vi "Replace GUIDs in Constants VI.vi"(8 "error in":errorcluster, 10 "guid map":map{string, string}(c390), 11 "VI in":refnum<vi>) -> (0 "error out":errorcluster, 3 "VI out":refnum<vi>)   [LabVIEW 2020, in "Utility.lvlib"]
uses:
  Utility.lvlib
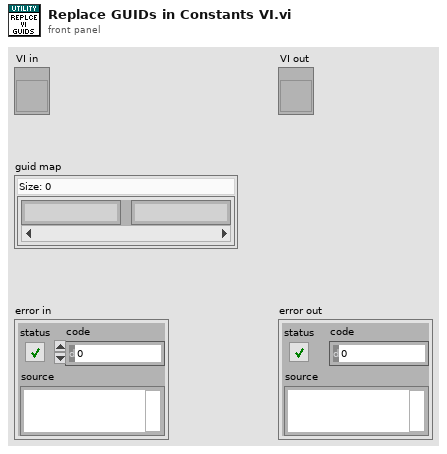
[diagram p1: front panel]
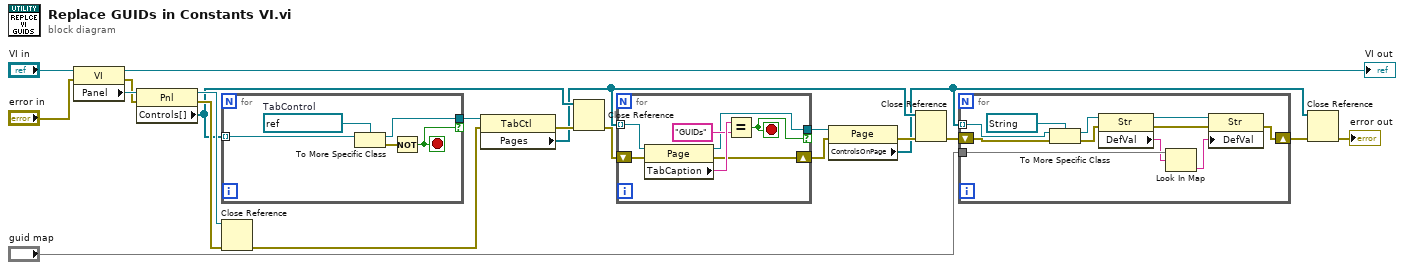
[diagram p0: block diagram]
diagram:
  n1 = property class="VI"(reference="VI in", error in="error in") -> (reference out=→"VI out":refnum<vi>, error out=w15:errorcluster, "Panel"=w19:refnum<vi>)
  n2 = property class="Pnl"(reference=w19, error in=w15) -> (reference out=w13:refnum<vi>, error out=w14:errorcluster, "Controls[]"=w5:refnum<vi>[])
  n3 = for {
    tunnel: w5 -> [w26] mode=indexing
    tunnel: [w24] -> w20 if=w22
    stop <- w22 stop-if-true
    w25 = refnum<vi> refnum  # TabControl
    n4 = To More Specific Class(target class=w25, reference=w26) -> (specific class reference=w24:refnum<vi>, error out=w23:errorcluster)  [unwired: 1 in]
    n5 = Not(x=w23) -> (.not. x?=w22:bool)
  }
  n6 = Close Reference(reference=w13, error in (no error)=w14) -> (error out=w12:errorcluster)
  n7 = property class="TabCtl"(reference=w20, error in=w12) -> (error out=w11:errorcluster, "Pages"=w3:refnum<vi>[])  [unwired: 1 out]
  n8 = Close Reference(reference=w5, error in (no error)=w11) -> (error out=w6:errorcluster)
  n9 = for {
    tunnel: w3 -> [w33] mode=indexing
    tunnel: [w30] -> w21 if=w29
    shift-right: [w27] -> w10
    shift-left: w6 -> [w28]
    stop <- w29 stop-if-true
    n10 = property class="Page"(reference=w33, error in=w28) -> (reference out=w30:refnum<vi>, error out=w27:errorcluster, "TabCaption"=w32:string)
    n11 = Equal?(x=w32, y="GUIDs") -> (x = y?=w29:bool)
  }
  n12 = property class="Page"(reference=w21, error in=w10) -> (error out=w9:errorcluster, "ControlsOnPage"=w1:refnum<vi>[])  [unwired: 1 out]
  n13 = Close Reference(reference=w3, error in (no error)=w9) -> (error out=w4:errorcluster)
  n14 = for {
    tunnel: w1 -> [w44] mode=indexing
    shift-right: [w34] -> w8
    shift-left: w4 -> [w40]
    tunnel: "guid map" -> [w39]
    n15 = To More Specific Class(target class=refnum<vi> refnum ("GUID.Import Frames"), reference=w44, error in=w40) -> (specific class reference=w42:refnum<vi>, error out=w41:errorcluster)
    n16 = property class="Str"(reference=w42, error in=w41) -> (reference out=w36:refnum<vi>, error out=w37:errorcluster, "DefVal"=w38:string)
    n17 = Look In Map(map=w39, key=w38) -> (value=w35:string)  [unwired: 1 in, 1 out]
    n18 = property class="Str"(reference=w36, error in=w37, "DefVal"=w35) -> (error out=w34:errorcluster)  [unwired: 1 out]
  }
  n19 = Close Reference(reference=w1, error in (no error)=w8) -> (error out=→"error out":errorcluster)
